vi "GetInstancePath.vi"(8 "error in (no error)":errorcluster, 11 "CLabVIEWItemVIM in":refnum<class "CLabVIEWItemVIM.lvclass">) -> (0 "error out":errorcluster, 1 "Instance path":string, 3 "CLabVIEWItemVIM out":refnum<class "CLabVIEWItemVIM.lvclass">)   [LabVIEW 2020, in "LabVIEWFiles.lvlib" / "CLabVIEWItemVIM.lvclass"]
uses:
  CLabVIEWItemVIM.lvclass
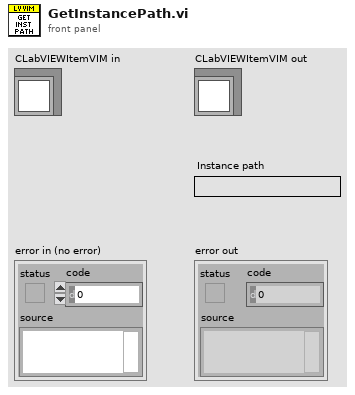
[diagram p1: front panel]
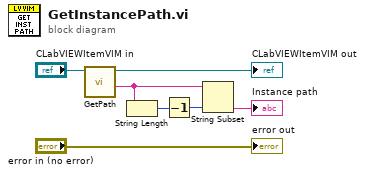
[diagram p0: block diagram]
diagram:
  n1 = call-dynamic "GetPath.vi"("CLabVIEWItem in"="CLabVIEWItemVIM in") -> ("Path"=w4:string, "CLabVIEWItem out"=→"CLabVIEWItemVIM out":refnum<class "CLabVIEWItemVIM.lvclass">)  [unwired: 8 in, 1 out]
  n2 = String Length(string=w4) -> (length=w3:i32)
  n3 = Decrement(x=w3) -> (x-1=w2:i32)
  n4 = String Subset(string=w4, length (rest)=w2) -> (substring=→"Instance path":string)  [unwired: 1 in]
  "error out" <- "error in (no error)"
